vi "niFPGA BFGroup Twiddle Table 32 U32 Inv.vi"(7 "address":fxp<+,5,5>) -> (4 "twid real":fxp<+/-,17,2> format="%.16g", 6 "twid imag":fxp<+/-,17,2> format="%.16g")   [LabVIEW 2017]
uses:
  <vilib>/rvi/FXPMathLib/basic elements/FxpDiscreteDelay/XNode/nifxpmath_DiscreteDelay.xnode
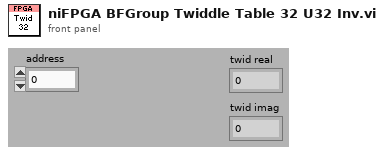
[diagram p1: front panel]
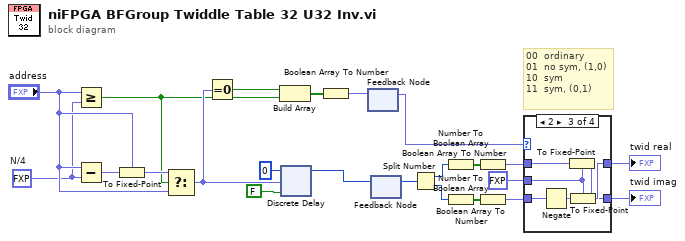
[diagram p0: block diagram]
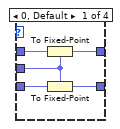
[diagram p2: hidden frame]
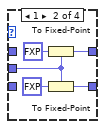
[diagram p3: hidden frame]
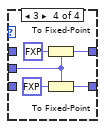
[diagram p4: hidden frame]
diagram:
  w3 = fxp<+,5,5> 16.0  # N/4
  # "00  ordinary\n01  no sym, (1,0)\n10  sym\n11  sym, (0,1)"
  n1 = Greater Or Equal?(x="address", y=w3) -> (x >= y?=w8:bool)
  n2 = Subtract(x="address", y=w3) -> (x-y=w18:fxp<+/-,6,6>)
  n3 = To Fixed-Point(fixed-point type="address", number=w18) -> (fixed-point=w17:fxp<+,5,5>)
  n4 = Select(t=w17, s=w8, f="address") -> (s? t:f=w11:fxp<+,5,5>)
  n5 = Equal To 0?(x=w11) -> (x = 0?=w7:bool)
  n6 = Build Array(w7, w8) -> (w9:bool[])
  n7 = xnode "Discrete Delay"("D"=u32 0, "n-1[0..15]"=w11, "enable"=FALSE) -> ("Q"=w10:u32)
  n8 = Boolean Array To Number(Boolean array=w9) -> (number=w6:fxp<+,2,2>)
  n9 = feedback-in #1(w6) -> ()
  n10 = feedback #1() -> (w5:fxp<+,2,2>)  [unwired: 1 out]
  n11 = feedback-in #2(w10) -> ()
  n12 = feedback #2() -> (w19:u32)  [unwired: 1 out]
  n13 = Split Number(x=w19) -> (hi(x)=w22:u16, lo(x)=w20:u16)
  n14 = Number To Boolean Array(number=w22) -> (Boolean array=w23:bool[])
  n15 = Number To Boolean Array(number=w20) -> (Boolean array=w21:bool[])
  n16 = Boolean Array To Number(Boolean array=w23) -> (number=w14:fxp<+/-,16,1>)
  n17 = Boolean Array To Number(Boolean array=w21) -> (number=w15:fxp<+/-,16,1>)
  n18 = case shown="2" w5 {
    tunnel: w14 -> [w28 _ w35 _]
    tunnel: [w27 w32 w38 w43] -> w2
    tunnel: w15 -> [w26 _ w39 _]
    tunnel: [w25 w30 w34 w41] -> w1
    tunnel: fxp<+/-,17,2> 0.0 ("fixed-point type") -> [w24 w29 w36 w40]
    frame 0, Default {
      n19 = To Fixed-Point(fixed-point type=w24, number=w28) -> (fixed-point=w27:fxp<+/-,17,2>)
      n20 = To Fixed-Point(fixed-point type=w24, number=w26) -> (fixed-point=w25:fxp<+/-,17,2>)
    }
    frame 1 {
      n21 = To Fixed-Point(fixed-point type=w29, number=fxp<+,1,1> 1.0 ("fixed-point type")) -> (fixed-point=w32:fxp<+/-,17,2>)
      n22 = To Fixed-Point(fixed-point type=w29, number=fxp<+,1,1> 0.0 ("fixed-point type")) -> (fixed-point=w30:fxp<+/-,17,2>)
    }
    frame 2 {
      n23 = Negate(x=w39) -> (-x=w37:fxp<+/-,17,2>)
      n24 = To Fixed-Point(fixed-point type=w36, number=w35) -> (fixed-point=w34:fxp<+/-,17,2>)
      n25 = To Fixed-Point(fixed-point type=w36, number=w37) -> (fixed-point=w38:fxp<+/-,17,2>)
    }
    frame 3 {
      n26 = To Fixed-Point(fixed-point type=w40, number=fxp<+,1,1> 0.0 ("fixed-point type")) -> (fixed-point=w43:fxp<+/-,17,2>)
      n27 = To Fixed-Point(fixed-point type=w40, number=fxp<+,1,1> 1.0 ("fixed-point type")) -> (fixed-point=w41:fxp<+/-,17,2>)
    }
  }
  "twid real" <- w2
  "twid imag" <- w1
